vi "Network Stream Image Target.vi"() -> ()   [LabVIEW 2013]
uses:
  <vilib>/dex/Stream Element Allocation Mode.ctl
  <vilib>/vision/Avi.llb/IMAQ AVI2 Codec Path.ctl
panel:
  in  "AVI fps":u32=5
  out "Codec Chosen":string="Motion JPEG (NI Vision)"
  out "error out":errorcluster
  out "Images in Queue":i32
  out "Codec Names":string[](array[string])
  in  "Codec Index":i32=1
  in  "Stop":bool
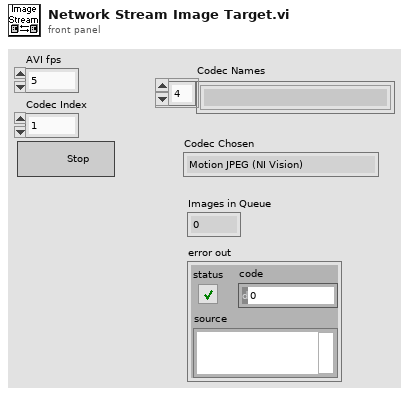
[diagram p1: front panel]
types:
  T1 = typedef "IMAQ AVI2 Codec Path.ctl" = u32
  T2 = typedef "Stream Element Allocation Mode.ctl" = u32
  T3 = typedef "Image Type" = u32
  T4 = typedef "IMAQ Image.ctl" = refnum<image>
  T5 = typedef "IMAQ AVI2 Refnum.ctl" = refnum<k20>
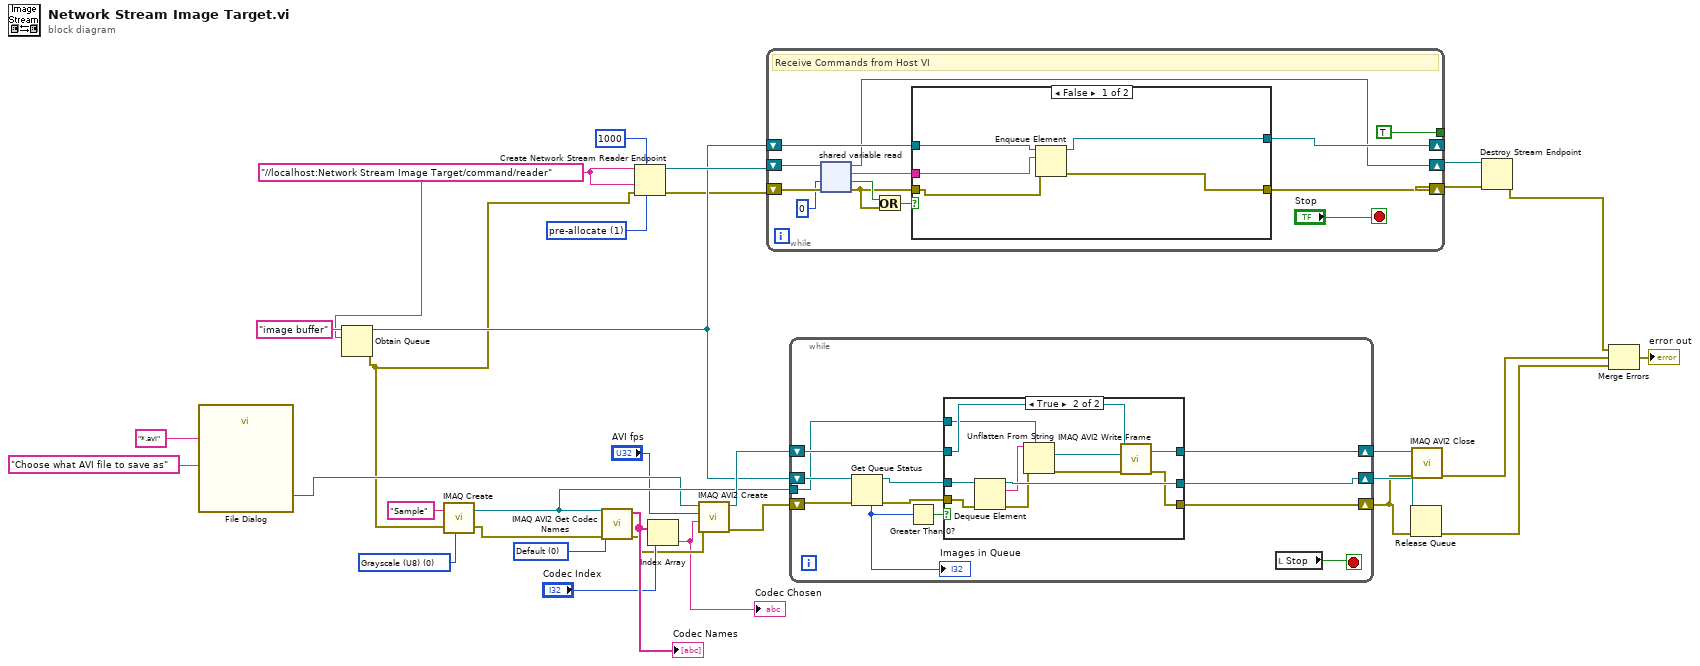
[diagram p0: block diagram]
diagram:
  w25 = T1 0 items=["Default", "System", "Built in Vision"] ("Codec Source")
  w28 = T2 1 items=["allocate as needed", "pre-allocate"] ("element allocation mode")
  w30 = T3 0 items=["Grayscale (U8)", "Grayscale (I16)", "Grayscale (SGL)", "Complex (CSG)", "RGB (U32)", "HSL (U32)", "RGB (U64)", "Grayscale (U16)"] ("Image Type")
  w15 = "//localhost:Network Stream Image Target/command/reader" ("reader url")
  n1 = call "File Dialog"("prompt"="Choose what AVI file to save as", "pattern (all files)"="*.avi" ("pattern label")) -> ("selected path"=w14:path)  [unwired: 10 in, 3 out]
  n2 = Obtain Queue(name (unnamed)="image buffer", element data type=w15) -> (queue out=w20:refnum<queue>, error out=w10:errorcluster)  [unwired: 3 in, 1 out]
  n3 = call "IMAQ Create"("Image Name"="Sample", "Image Type"=w30, "error in (no error)"=w10) -> ("New Image"=w16:T4, "error out"=w13:errorcluster)  [unwired: 2 in]
  n4 = call "IMAQ AVI2 Get Codec Names"("error in (no error)"=w13, "Codec Source"=w25, "Image"=w16) -> ("error out"=w12:errorcluster, "Codec Names"=w24:string[])  [unwired: 7 in]
  "Codec Names" <- w24
  n5 = Create Network Stream Reader Endpoint(6:w28, 7:1000 ("reader buffer size"), 8:w10, 9:w15, 11:w15) -> (0:w18:errorcluster, 3:w32:refnum<k21>)  [unwired: 2 in]
  n6 = Index Array(array=w24, index="Codec Index") -> (element=w2:string)
  "Codec Chosen" <- w2
  n7 = call "IMAQ AVI2 Create"("error in (no error)"=w12, "Codec"=w2, "Frames Per Second"="AVI fps", "AVI Path"=w14) -> ("error out"=w11:errorcluster, "AVI Refnum"=w21:T5)  [unwired: 6 in]
  n8 = while "Host->Target Command Reader" {
    shift-right: [w42] -> w27
    shift-left: w18 -> [w45]
    shift-right: [w33] -> w26
    shift-left: w32 -> [w44]
    tunnel: [TRUE] -> _
    shift-right: [w35] -> _
    shift-left: w20 -> [w36]
    stop <- "Stop" stop-if-true
    # "Receive Commands from Host VI"
    n9 = shared-variable-read(w44, w45, 0 ("timeout ms")) -> (w33:refnum<k21>, w39:errorcluster, w41:bool, w37:string)
    n10 = Or(x=w41, y=w39) -> (x .or. y?=w40:bool)
    n11 = case shown="False" w40 {
      tunnel: w39 -> [w47 w52]
      tunnel: [w46 w52] -> w42
      tunnel: w37 -> [w48 _]
      tunnel: w36 -> [w50 w51]
      tunnel: [w49 w51] -> w35
      frame False {
        n12 = Enqueue Element(queue=w50, element=w48, error in (no error)=w47) -> (queue out=w49:refnum<queue>, error out=w46:errorcluster)  [unwired: 1 in, 1 out]
      }
      frame True {
      }
    }
  }
  n13 = while {
    shift-right: [w59] -> w19
    shift-left: w21 -> [w61]
    shift-right: [w58] -> w17
    shift-left: w20 -> [w64]
    tunnel: w16 -> [w57]
    shift-right: [w53] -> w9
    shift-left: w11 -> [w55]
    stop <- w56 stop-if-true
    n14 = Get Queue Status(queue=w64, error in (no error)=w55) -> (queue out=w60:refnum<queue>, error out=w54:errorcluster, # elements in queue=w63:i32)  [unwired: 1 in, 5 out]
    "Images in Queue" <- w63
    n15 = Greater Than 0?(x=w63) -> (x > 0?=w62:bool)
    n16 = case shown="True" w62 {
      tunnel: w61 -> [w67 w74]
      tunnel: w60 -> [w66 w78]
      tunnel: [w67 w77] -> w59
      tunnel: [w66 w76] -> w58
      tunnel: w57 -> [_ w72]
      tunnel: w54 -> [w65 w71]
      tunnel: [w65 w68] -> w53
      frame False {
      }
      frame True {
        n17 = Dequeue Element(queue=w78, error in (no error)=w71) -> (queue out=w76:refnum<queue>, element=w75:string, error out=w70:errorcluster)  [unwired: 1 in, 1 out]
        n18 = Unflatten From String(type=w72, binary string=w75, error in (no error)=w70) -> (value=w73:T4, error out=w69:errorcluster)  [unwired: 2 in, 1 out]
        n19 = call "IMAQ AVI2 Write Frame"("error in (no error)"=w69, "Image"=w73, "AVI Refnum"=w74) -> ("error out"=w68:errorcluster, "AVI Refnum (duplicate)"=w77:T5)  [unwired: 6 in, 1 out]
      }
    }
    n20 = local read "Stop"() -> (w56:bool)
  }
  n21 = Release Queue(queue=w17, error in (no error)=w9) -> (error out=w6:errorcluster)  [unwired: 1 in, 2 out]
  n22 = call "IMAQ AVI2 Close"("error in (no error)"=w9, "AVI Refnum"=w19) -> ("error out"=w7:errorcluster)  [unwired: 9 in]
  n23 = Destroy Stream Endpoint(8:w27, 11:w26) -> (0:w8:errorcluster)
  n24 = Merge Errors(w8, w7, w6) -> (→"error out":errorcluster)
